vi "Stop Core.vi"(10 "final error code":i32, 11 "Operator UI Actor in":refnum<class "Measurement UI.lvclass">) -> (3 "Operator UI Actor out":refnum<class "Measurement UI.lvclass">)   [LabVIEW 2015, in "Measurement UI.lvlib" / "Measurement UI.lvclass"]
uses:
  Measurement UI.lvclass
  User Interface/UI.lvclass
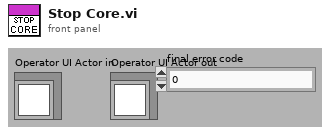
[diagram p1: front panel]
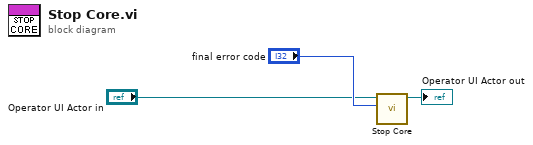
[diagram p0: block diagram]
diagram:
  n1 = call-parent "Stop Core.vi"("final error code"="final error code", "UI in"="Operator UI Actor in") -> ("UI out"=→"Operator UI Actor out":refnum<class "Measurement UI.lvclass">)  [unwired: 9 in]
